vi "PS35_GetReadError.vi"(1 "Control unit ID":i32=1 min=1 max=10) -> (0 "Read error":i32)   [LabVIEW 2020]
doc: "PS35_GetReadError.vi, created: 03.03.2009 alex; last change: 22.10.2019 alex;\n\n<B>FUNCTION:</B> \n\nRead error code of the last read function (PS35_Get...).\n----------------------------------------------------------------------------------------\n<B>INPUT:</B>\n[I32] <B>Control unit ID:</B> control unit index. (Default=1, Range=1...10) \n----------------------------------------------------------------------------------------\n<B>OUTPUT:</B>\n[I32] <B>Read error:</B> error code of the last read function.\n 0 - function was successful (no error),\n-1 - function error,\n-2 - communication error,\n-3 - syntax error,\n-4 - axis in wrong state.\n----------------------------------------------------------------------------------------\n<B>SUB-VIs:</B>\n----------------------------------------------------------------------------------------\n<B>EXT-Calls:</B>\nps35.dll (V2.01)\n----------------------------------------------------------------------------------------"
uses:
  ps35.dll
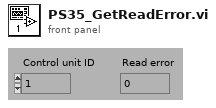
[diagram p1: front panel]
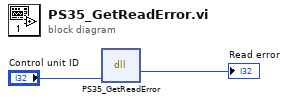
[diagram p0: block diagram]
diagram:
  n1 = dll-call lib="C:/GEECS/Developers Version/source/Device Drivers/OwiSoft_PS35/OWISoftOEM/ps35/labview/lv82/ps35.dll" fn="PS35_GetReadError"("Index"="Control unit ID") -> ("Rückgabetyp"=→"Read error":i32)  [unwired: 4 in, 2 out]
